vi "demo_idn.vi"() -> ()   [LabVIEW 2017]
panel:
  out "IDN":string
  in  "name":string="mrx-t4"
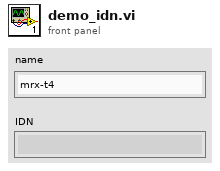
[diagram p1: front panel]
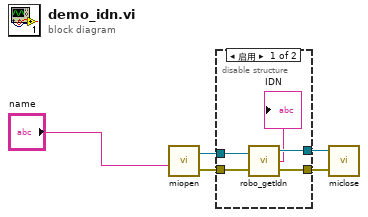
[diagram p0: block diagram]
diagram:
  n1 = call "miopen.vi"("name"="name") -> ("错误输出"=w2:errorcluster, "连接ID"=w5:refnum<k5>)  [unwired: 3 in]
  n2 = disable-structure shown="启用" {
    disable-tunnel: w5 -> [w10 w12]
    disable-tunnel: [w9 w12] -> w4
    disable-tunnel: [w8 w11] -> w3
    disable-tunnel: w2 -> [w7 w11]
    frame Enabled {
      n3 = call "robo_getIdn.vi"("连接ID"=w10, "错误输入（无错误）"=w7) -> ("连接ID输出"=w9:refnum<k5>, "读取缓冲区"=→"IDN":string, "错误输出"=w8:errorcluster)
    }
    frame Disabled {
    }
  }
  n4 = call "miclose.vi"("错误输入（无错误）"=w3, "连接ID"=w4) -> ()  [unwired: 1 out]
